vi "Add AI Channels.vi"(8 "error in (no error)":errorcluster, 10 "Channels":u8, 11 "Device Item Ref in":T1 format="%.0x") -> (0 "error out":errorcluster, 3 "Parent Ref out":T1 format="%.0x")   [LabVIEW 2021, in "DAQ Analog InOut System Explorer.lvlib"]
doc: "Add an Analog Output channel based on the physical channel specified"
uses:
  DAQ Analog InOut System Explorer.lvlib
  <vilib>/NI VeriStand/Custom Device API/Custom Device Item Ref.ctl
  <vilib>/NI VeriStand/Custom Device API/Custom Device Channel.ctl
  <vilib>/NI VeriStand/Custom Device API/Custom Device Channel Type.ctl
  <vilib>/NI VeriStand/Custom Device Tools/Custom Device Utility Library/NI VeriStand - Search for Item by Name.vi
  <vilib>/NI VeriStand/Custom Device API/Custom Device API.lvlib
  <vilib>/NI VeriStand/Custom Device Tools/Custom Device Utility Library/Custom Device Utility Library.lvlib
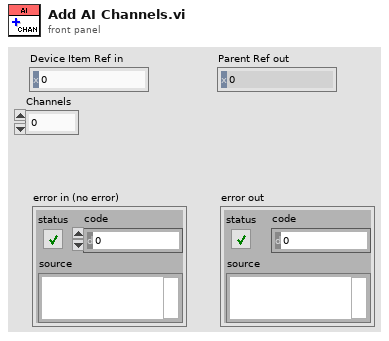
[diagram p1: front panel]
types:
  T1 = typedef "Custom Device API.lvlib/Custom Device Item Ref.ctl" = u64
  T2 = typedef "Custom Device API.lvlib/Custom Device Channel.ctl" = cluster{"Type":T3, "Units":string, "Default Value":dbl, "Faultable":bool, "Scalable":bool}
  T3 = typedef "Custom Device API.lvlib/Custom Device Channel Type.ctl" = enum16{"Input", "Output"}
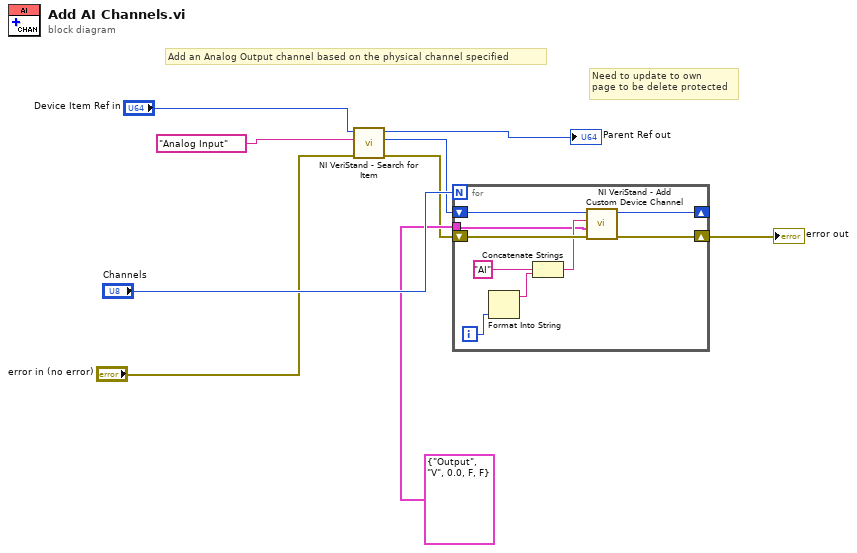
[diagram p0: block diagram]
diagram:
  # "Need to update to own\npage to be delete protected"
  # "Add an Analog Output channel based on the physical channel specified"
  n1 = call-poly <vilib>:"NI VeriStand - Search for Item.vi"("error in"="error in (no error)", "Item Name"="Analog Input" ("format string"), "Section Ref in"="Device Item Ref in") -> ("error out"=w1:errorcluster, "Item Ref"=w3:T1, "Section Ref out"=→"Parent Ref out":T1)  [unwired: 5 in, 1 out]
  n2 = for {
    N: "Channels" -> [_]
    shift-right: [w15] -> w8
    shift-left: w1 -> [w17]
    shift-right: [w16] -> _
    shift-left: w3 -> [w18]
    tunnel: T2 {"Type"=enum."Output", "Units"="V", "Default Value"=0.0, "Faultable"=FALSE, "Scalable"=FALSE} ("Channel") -> [w10]
    i -> [w13]
    n3 = Format Into String(w13) -> (resulting string=w12:string)  [unwired: 3 in, 1 out]
    n4 = Concatenate Strings("AI", w12) -> (w11:string)
    n5 = call <vilib>:"NI VeriStand - Add Custom Device Channel.vi"("error in (no error)"=w17, "Channel"=w10, "Channel Name"=w11, "Parent Ref in"=w18) -> ("error out"=w15:errorcluster, "Parent Ref out"=w16:T1)  [unwired: 4 in, 2 out]
  }
  "error out" <- w8
